vi "Get Plugin Thread Name.vi"(8 "error in (no error)":errorcluster, 9 "Thread ID":u8, 10 "Plugin ID":u8, 11 "Logging Thread in":refnum<class "Logging Thread.lvclass">) -> (0 "error out":errorcluster, 2 "thread name":string, 3 "Logging Thread out":refnum<class "Logging Thread.lvclass">)   [LabVIEW 2019, in "DSF Core.lvlib" / "Logging Thread.lvclass"]
uses:
  Logging Thread.lvclass
  Logging Thread.lvclass/Logging Thread.ctl
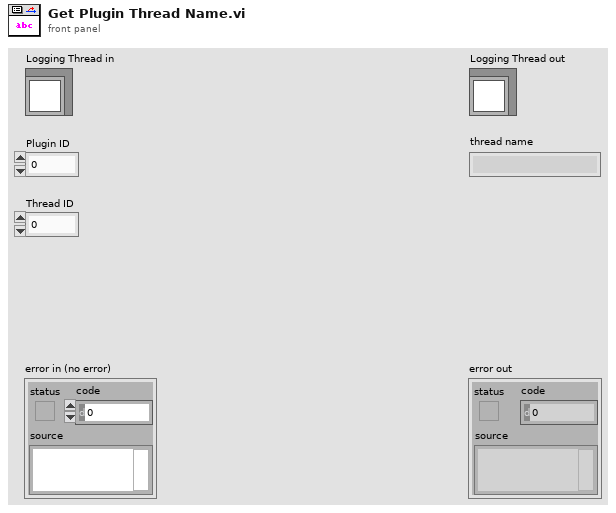
[diagram p1: front panel]
types:
  T1 = typedef "DSF Core.lvlib/Logging Thread.lvclass/Plugin Data.ctl" = cluster{"thread names":string[]}
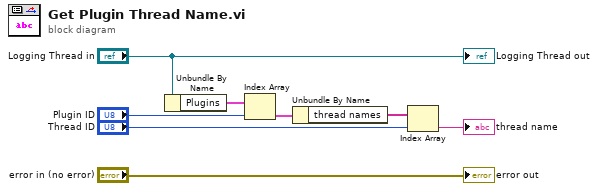
[diagram p0: block diagram]
diagram:
  n1 = Unbundle By Name("Logging Thread in") -> ("Plugins"=w7:T1[])
  n2 = Index Array(array=w7, index="Plugin ID") -> (element=w6:T1)
  n3 = Unbundle By Name(w6) -> ("thread names"=w5:string[])
  n4 = Index Array(array=w5, index="Thread ID") -> (element=→"thread name":string)
  "error out" <- "error in (no error)"
  "Logging Thread out" <- "Logging Thread in"
